vi "Op-Amp Test System.vi"() -> ()   [LabVIEW 2019]
uses:
  <vilib>/Utility/error.llb/DialogType.ctl
  <vilib>/VirtualBench/_DMM Configure Measurement2.vi
  <vilib>/VirtualBench/_PS Configure Voltage Output0.vi
  <vilib>/VirtualBench/_FGEN Configure Standard Waveform14.vi
  <vilib>/VirtualBench/_FGEN Configure Standard Waveform4.vi
  <vilib>/VirtualBench/_MSO Configure Analog Channel28.vi
  <vilib>/VirtualBench/_MSO Configure Timing12.vi
  <vilib>/VirtualBench/_MSO Configure Digital Edge Trigger0.vi
  <vilib>/VirtualBench/_MSO Configure Analog Edge Trigger0.vi
  <vilib>/VirtualBench/_MSO Configure Digital Pattern Trigger0.vi
  <vilib>/VirtualBench/_MSO Configure Analog Channel29.vi
  <vilib>/VirtualBench/VirtualBench.lvlib
  <vilib>/DigilentWF/DigilentWF.lvlib
panel:
  out "测试进度":u8(slide)=100 caption="Testing..." scale=0.0..100.0
  in  "开始测试":bool caption="Start"
  out "Slew Rate(V/us)":dbl=0.5925925925925918 format="%#.2f"
  out "Iin+(mA)":dbl=0.032890531941645075 format="%#.2g"
  out "Voffset(mV)":dbl=0.00017364742031570723 format="%#.2f"
  out "Iin-(mA)":dbl=0.032890531941645075 format="%#.2g"
  in  "图表选项卡":enum32{"Time Domain", "Frequency Domain"}(tab)
  out "Time Domain":waveform(dbl)(graph)={"t0"=timestamp(3648703829.272387 s since 1904-01-01), "dt"=5e-06, "Y"=[1.4814814814814814, 1.522633744855967, 1.522633744855967, 1.522633744855967, 1.522633744855967, -1.4814814814814814, -1.4814814814814814, -1.4814814814814814, -1.4814814814814814, -1.4814814814814814, 1.4814814814814814, 1.4814814814814814, 1.522633744855967, 1.522633744855967, 1.522633744855967, -1.4814814814814814, -1.4814814814814814, -1.4814814814814814, -1.522633744855967, -1.4814814814814814, 1.4814814814814814, 1.4814814814814814, 1.522633744855967, 1.522633744855967, 1.4814814814814814, -1.4814814814814814, -1.4814814814814814, -1.4814814814814814, -1.4814814814814814, -1.4814814814814814, 1.522633744855967, 1.4814814814814814, 1.522633744855967, 1.4814814814814814, 1.522633744855967, -1.4814814814814814, -1.4814814814814814, -1.4814814814814814, -1.4814814814814814, -1.4814814814814814, 1.4814814814814814, 1.522633744855967, 1.522633744855967, 1.522633744855967, 1.4814814814814814, -1.4814814814814814, -1.4814814814814814, -1.4814814814814814, -1.4814814814814814, -1.4814814814814814, 1.522633744855967], "attributes"=variant("NI_ChannelName"=variant(string "mso/1"), "NI_UnitDescription"=variant(string "Volts"))}
  out "Amplitude-frequency":cluster{dbl[], dbl[]}(graph)={[1000.0, 50000.0, 100000.0, 150000.0, 200000.0, 250000.0, 300000.0, 350000.0, 400000.0, 450000.0, 500000.0, 550000.0, 600000.0, 650000.0, 700000.0, 750000.0, 800000.0, 850000.0, 900000.0, 950000.0, 1000000.0], [-0.043499224382493214, -0.07910564758937852, -0.05855677171822875, -0.12520052009093197, -0.0701265456021912, -0.03557595242825849, -0.039394402754777826, 0.019459305615298683, -0.20860878085057782, -0.6531346266811084, -1.6767532340802709, -2.545389095285617, -3.45499166219188, -4.165947530618234, -5.023851452790434, -5.691370407236383, -6.452267174495198, -6.919081220388349, -7.501631061654676, -8.082809544588587, -8.419860804310309]} caption="Amplitude-frequency characteristic"
  out "PSRR(dB)":dbl=139.0596904318624 format="%#.1f"
  out "KCMRR(dB)":dbl=128.17369955860022 format="%#.1f"
  out "Iin_mean(mA)":dbl=0.032890531941645075 format="%#.2g"
  out "Iin_bias(mA)":dbl format="%#.5g"
  out "K0(dB)":dbl=131.53455047796112 format="%#.1f"
  in  "测试参数选项卡":T1(tab)=enum."Slew Rate"
  in  "Current PWS":T2={"PWS Channel"="VB8012-3126A15/ps/+25V", "Voltage Level (V)"=10.0, "Current Limit (A)"=0.05} {"Voltage Level (V)" min=0.0 max=12.0}
  in  "DC Offset(V)":dbl=1.0 caption="DC Offset" format="%#_13g"
  in  "Waveform Function":enum16{"Sine", "Square", "Triangle/Ramp", "DC"}(ring)=enum."DC"
  in  "CMRR PWS 2":T3={"PWS Channel 2"="VB8012-3126A15/ps/-25V", "Voltage Level (V)"=[-9.5, -8.5], "Current Limit (A)"=0.05} {"Voltage Level (V)" min=-12.0 max=0.0}
  in  "CMRR PWS1":T4={"PWS Channel 1"="VB8012-3126A15/ps/+25V", "Voltage Level (V)"=[9.5, 10.5], "Current Limit (A)"=0.05} {"Voltage Level (V)" min=0.0 max=12.0}
  in  "PSRR PWS":T5={"PWS Channel"="VB8012-3126A15/ps/+25V", "Voltage Level (V)"=[9.5, 10.0], "Current Limit (A)"=0.05} {"Voltage Level (V)" min=0.0 max=12.0}
  in  "Slew Rate PWS":T2={"PWS Channel"="VB8012-3126A15/ps/+25V", "Voltage Level (V)"=10.0, "Current Limit (A)"=0.05} {"Voltage Level (V)" min=0.0 max=12.0}
  in  "Frequency":dbl=20000.0 format="%#_13g"
  in  "Slewrate Waveform":enum16{"Sine", "Square", "Triangle/Ramp", "DC"}(ring)=enum."Square" caption="Waveform Function"
  in  "Amplitude":dbl=3.0 format="%#_13g"
  in  "DC Offset":dbl format="%#_13g"
  in  "Channel":tag="VB8012-3126A15/mso/1"
  in  "Vertical Range":dbl=3.0 format="%#_13g"
  in  "Trigger Type":T6(tab)
  in  "Digital Trigger Source":tag="mso/d0" caption="Trigger Source (no change)"
  in  "Edge":i32(ring) caption="Trigger Slope (no change)" items=["Rising", "Falling", "Either"]
  in  "Level (V)":dbl=0.4 format="%0.2f"
  in  "Hysteresis (V)":dbl=0.17
  in  "Analog Trigger Source":tag="VB8012-3126A15/mso/1" caption="Trigger Source (no change)"
  in  "Slope":i32(ring) caption="Trigger Slope (no change)" items=["Rising", "Falling", "Either"]
  in  "Pattern Trigger Source":tag="mso/d0:7" caption="Trigger Source (no change)"
  in  "Trigger Pattern":string="1R0XX1X0" caption="Trigger Pattern (no change)"
  in  "BW PWS":T2={"PWS Channel"="VB8012-3126A15/ps/+25V", "Voltage Level (V)"=10.0, "Current Limit (A)"=0.05} {"Voltage Level (V)" min=0.0 max=12.0}
  in  "Slewrate Waveform":enum16{"Sine", "Square", "Triangle/Ramp", "DC"}(ring) caption="Waveform Function"
  in  "Amplitude":dbl=2.0 format="%#_13g"
  in  "DC Offset":dbl format="%#_13g"
  in  "Vertical Range":dbl=3.0 format="%#_13g"
  in  "Channel":tag="VB8012-3126A15/mso/1"
  in  "Trigger Type":T6(tab)
  in  "Digital Trigger Source":tag="mso/d0" caption="Trigger Source (no change)"
  in  "Edge":i32(ring) caption="Trigger Slope (no change)" items=["Rising", "Falling", "Either"]
  in  "Analog Trigger Source":tag="mso/1" caption="Trigger Source (no change)"
  in  "Slope":i32(ring) caption="Trigger Slope (no change)" items=["Rising", "Falling", "Either"]
  in  "Level (V)":dbl format="%0.2f"
  in  "Hysteresis (V)":dbl=0.17
  in  "Pattern Trigger Source":tag="mso/d0:7" caption="Trigger Source (no change)"
  in  "Trigger Pattern":string="1R0XX1X0" caption="Trigger Pattern (no change)"
  in  "测试机台选择":tag="VB8012-3126A15"
  # "基于IECUBE-3839的运放自动化测试程序"
  # "硬件配置"
  # "DUT测试参数"
  # "设备选择"
  # "DUT测试结果"
  # "电源配置"
  # "函数发生器配置"
  # "电源配置"
  # "电源配置"
  # "电源配置"
  # "函数发生器配置"
  # "逻辑分析仪配置"
  # "Triggers immediately after MSO Run VI executes."
  # "电源配置"
  # "函数发生器配置"
  # "逻辑分析仪配置"
  # "Triggers immediately after MSO Run VI executes."
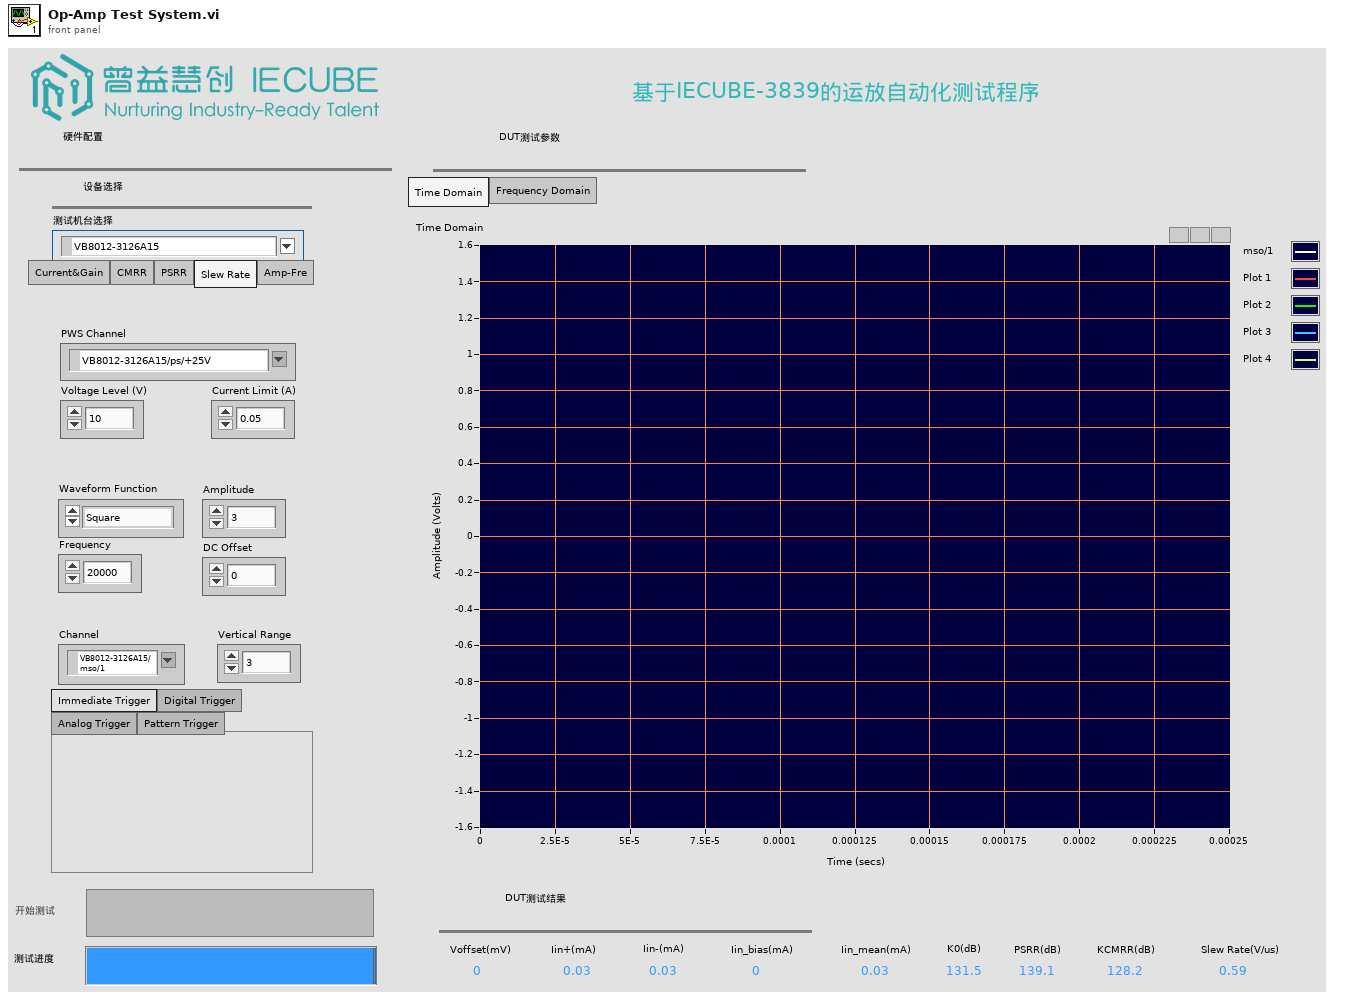
[diagram p1: front panel]
types:
  T1 = enum32{"Current&Gain", "CMRR", "PSRR", "Slew Rate", "Amp-Fre"}
  T2 = cluster{"PWS Channel":tag, "Voltage Level (V)":dbl, "Current Limit (A)":dbl}
  T3 = cluster{"PWS Channel 2":tag, "Voltage Level (V)":dbl[], "Current Limit (A)":dbl}
  T4 = cluster{"PWS Channel 1":tag, "Voltage Level (V)":dbl[], "Current Limit (A)":dbl}
  T5 = cluster{"PWS Channel":tag, "Voltage Level (V)":dbl[], "Current Limit (A)":dbl}
  T6 = enum32{"Immediate Trigger", "Digital Trigger", "Analog Trigger", "Pattern Trigger"}
  T7 = typedef "测试参数.ctl" = enum16{"Leakage Current", "Gain", "CMRR", "PSRR", "Slew Rate", "Amplitude-Frequency"}
  T8 = typedef "DialogType.ctl" = u16
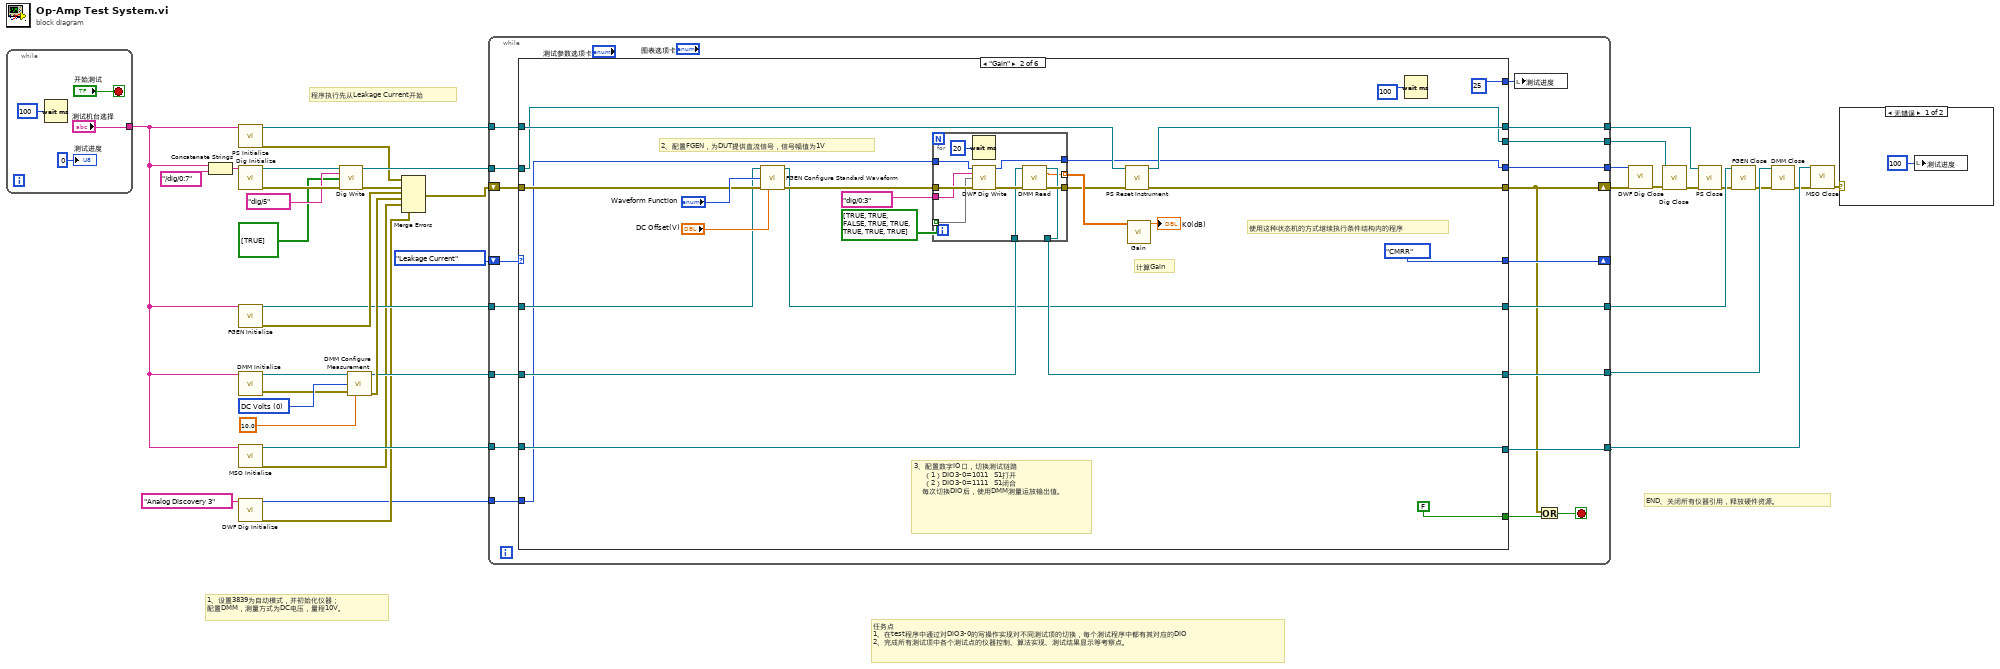
[diagram p0: block diagram]
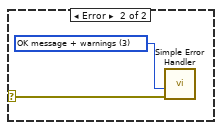
[diagram p2: hidden frame]
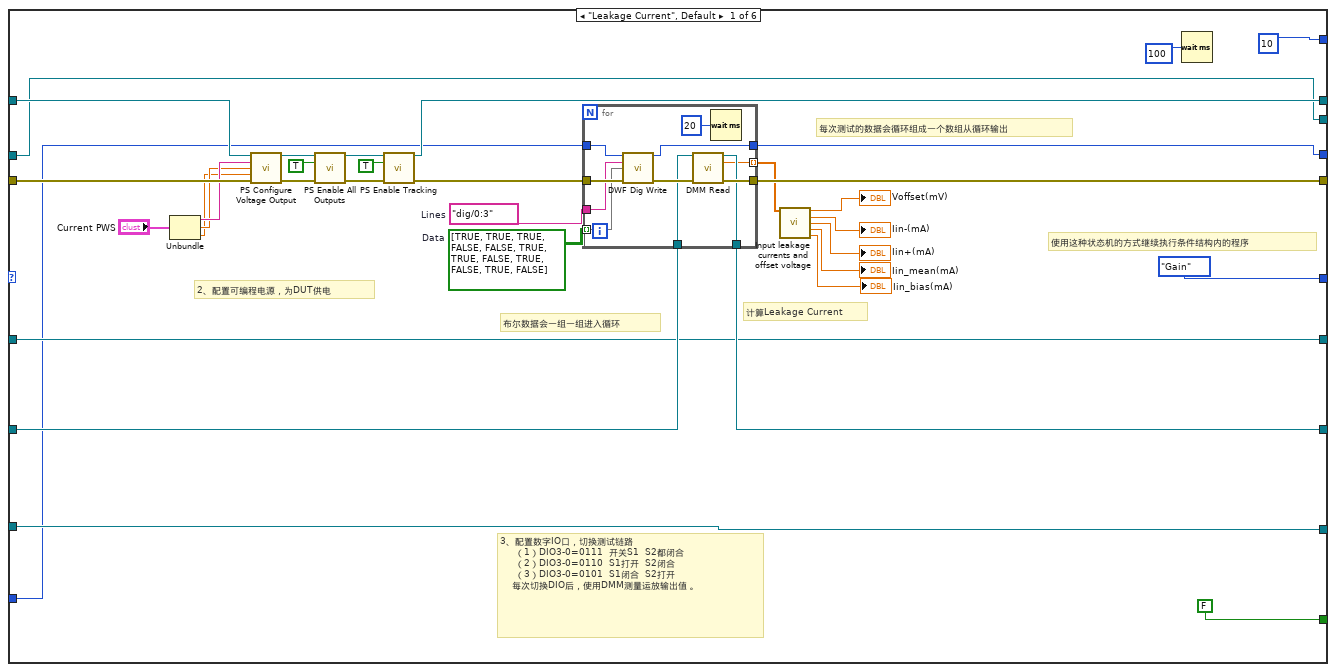
[diagram p3: hidden frame]
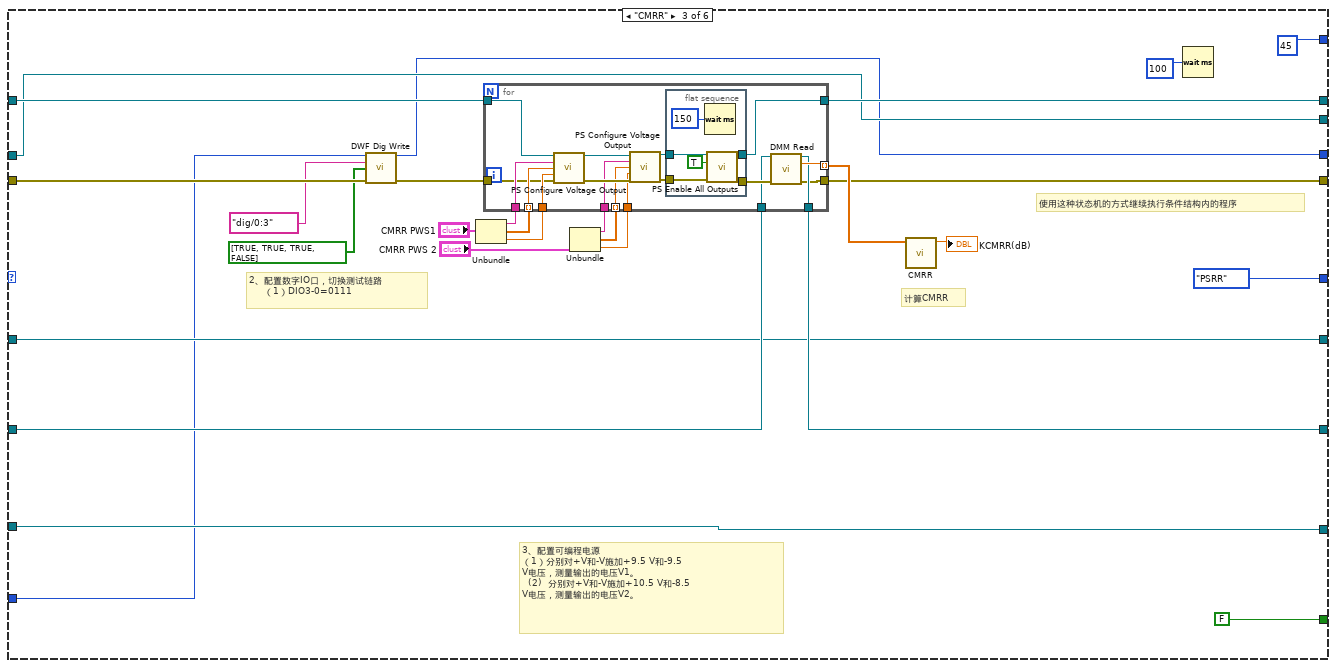
[diagram p4: hidden frame]
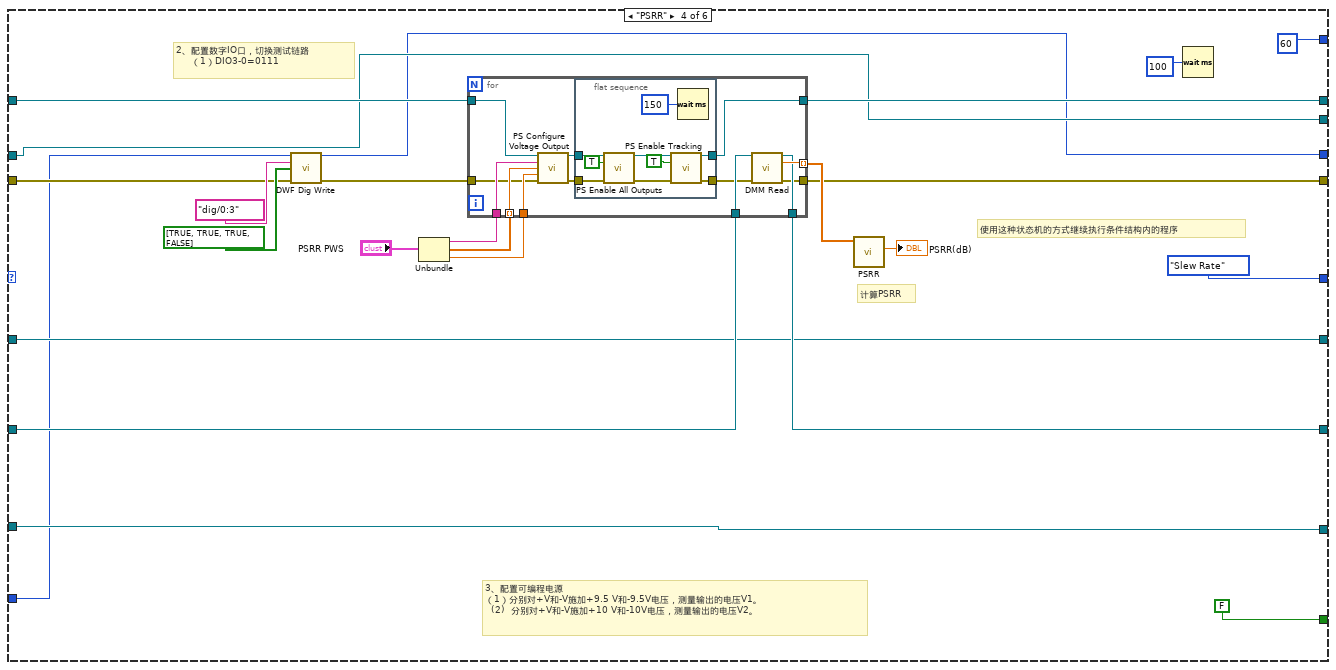
[diagram p5: hidden frame]
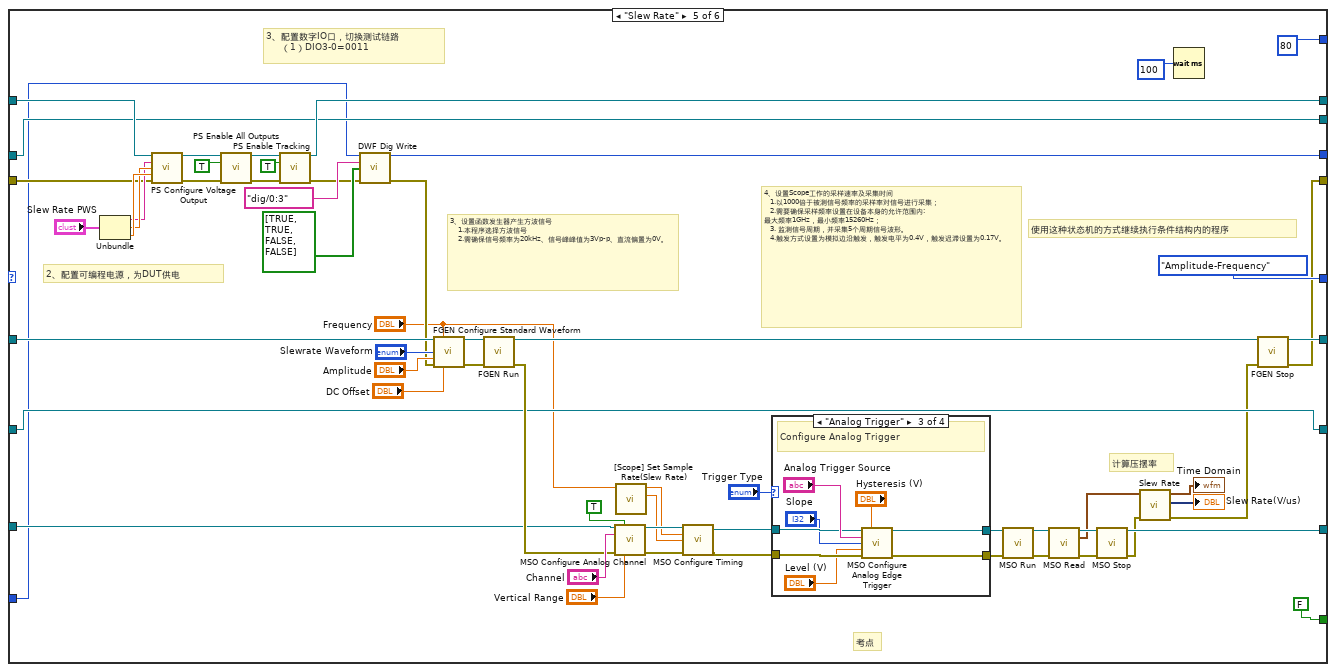
[diagram p6: hidden frame]
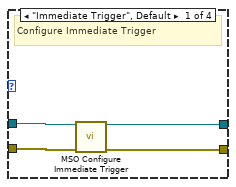
[diagram p7: hidden frame]
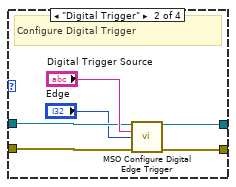
[diagram p8: hidden frame]
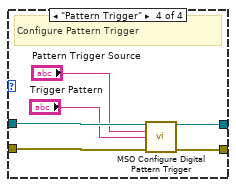
[diagram p9: hidden frame]
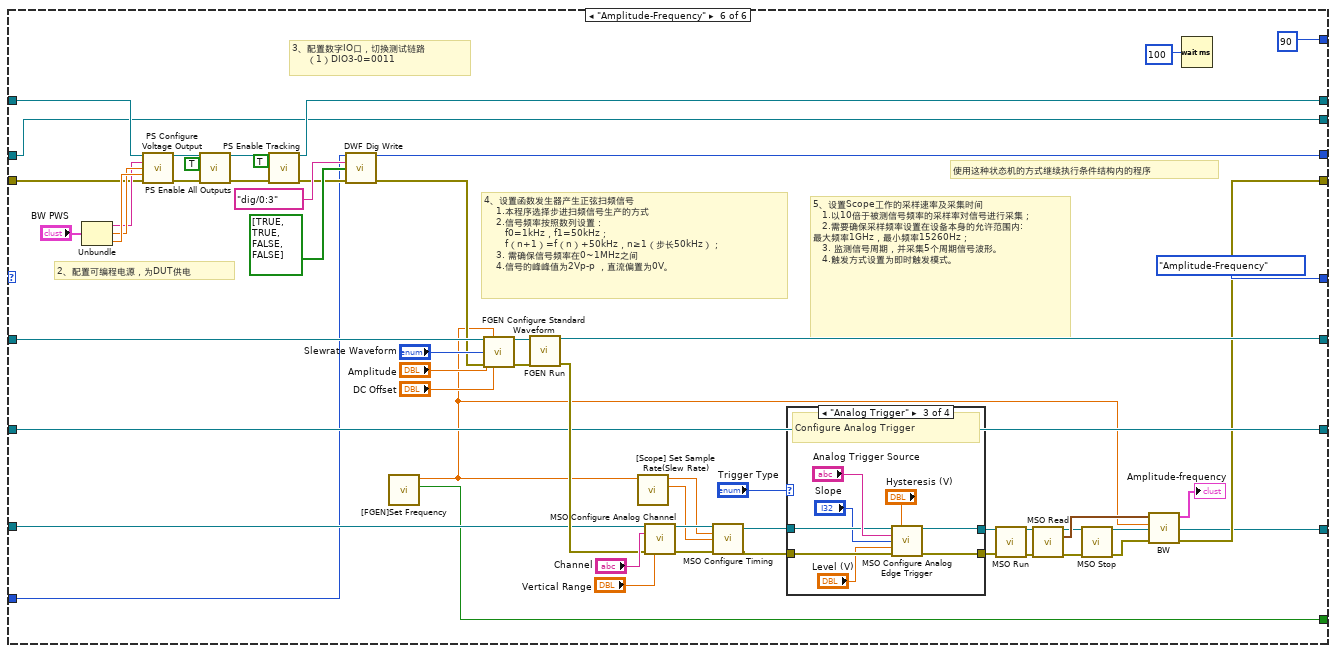
[diagram p10: hidden frame]
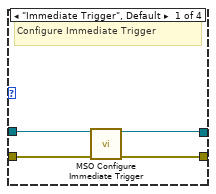
[diagram p11: hidden frame]
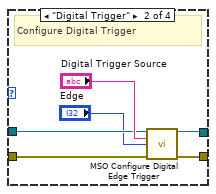
[diagram p12: hidden frame]
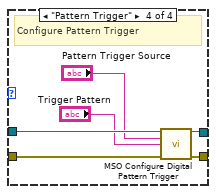
[diagram p13: hidden frame]
diagram:
  w29 = 0 items=["DC Volts", "AC Volts", "DC Current", "AC Current", "Resistance", "Diode"] ("Function")
  # "程序执行先从Leakage Current开始"
  # "任务点\n1、在test程序中通过对DIO3-0的写操作实现对不同测试项的切换，每个测试程序中都有其对应的DIO\n2、完成所有测试项中各个测试点的仪器控制、算法实现、测试结果显示等考察点。"
  # "END、关闭所有仪器引用，释放硬件资源。"
  # "1、设置3839为自动模式，并初始化仪器；\n配置DMM，测量方式为DC电压，量程10V。"
  n1 = while {
    tunnel: ["测试机台选择"] -> w16
    stop <- "开始测试" stop-if-true
    n2 = Wait (ms)(milliseconds to wait=u32 100 ("等待时间（毫秒）")) -> ()  [unwired: 1 out]
    "测试进度" <- u8 0 ("测试进度")
  }
  n3 = Concatenate Strings(w16, "/dig/0:7" ("字符串")) -> (w34:string)
  n4 = call <vilib>:"PS Initialize.vi"("Device Name"=w16) -> ("Instrument Handle Out"=w33:refnum<k21>, "Error Out"=w13:errorcluster)  [unwired: 13 in]
  n5 = call <vilib>:"Dig Initialize.vi"("Lines"=w34) -> ("Instrument Handle Out"=w39:refnum<k21>, "Error Out"=w38:errorcluster)  [unwired: 13 in]
  n6 = call <vilib>:"FGEN Initialize.vi"("Device Name"=w16) -> ("Instrument Handle Out"=w22:refnum<k21>, "Error Out"=w23:errorcluster)  [unwired: 13 in]
  n7 = call <vilib>:"DMM Initialize.vi"("Device Name"=w16) -> ("Instrument Handle Out"=w27:refnum<k21>, "Error Out"=w28:errorcluster)  [unwired: 13 in]
  n8 = call <vilib>:"MSO Initialize.vi"("Device Name"=w16) -> ("Instrument Handle Out"=w15:refnum<k21>, "Error Out"=w14:errorcluster)  [unwired: 13 in]
  n9 = call <vilib>:"DWF Dig Initialize.vi"("Device Name/Lines"="Analog Discovery 3") -> ("Instrument Handle Out"=w4:u32, "Error Out"=w5:errorcluster)  [unwired: 13 in]
  n10 = call <vilib>:"Dig Write.vi"("Instrument Handle In"=w39, "Lines"=tag "dig/5", "Data"=bool[] [TRUE], "Error In"=w38) -> ("Instrument Handle Out"=w32:refnum<k21>, "Error Out"=w12:errorcluster)  [unwired: 10 in]
  n11 = call-poly <vilib>:"DMM Configure Measurement.vi"("Instrument Handle In"=w27, "Function"=w29, "Error In"=w28, "Manual Range"=10.0) -> ("Instrument Handle Out"=w25:refnum<k21>, "Error Out"=w26:errorcluster)  [unwired: 10 in]
  n12 = Merge Errors(w13, w12, w23, w26, w14, w5) -> (w30:errorcluster)
  n13 = while {
    tunnel: w32 -> [w60]
    tunnel: w33 -> [w58]
    shift-right: [w59] -> _
    shift-left: 测试参数."Leakage Current" -> [w62]
    tunnel: w25 -> [w57]
    tunnel: [w56] -> w19
    shift-right: [w48] -> w2
    shift-left: w30 -> [w61]
    tunnel: [w55] -> w21
    tunnel: [w54] -> w20
    tunnel: w22 -> [w53]
    tunnel: [w52] -> w18
    tunnel: [w51] -> w17
    tunnel: w15 -> [w50]
    tunnel: w4 -> [w45]
    tunnel: [w44] -> w1
    stop <- w46 stop-if-true
    n14 = case shown="\"Gain\"" w62 {
      tunnel: w61 -> [w82 w122 w149 w198 w263 w344]
      tunnel: w60 -> [w65 w110 w145 w197 w243 w326]
      tunnel: [测试参数."Gain" 测试参数."CMRR" 测试参数."PSRR" 测试参数."Slew Rate" 测试参数."Amplitude-Frequency" 测试参数."Amplitude-Frequency"] -> w59
      tunnel: w58 -> [w80 w113 w167 w215 w262 w343]
      tunnel: w57 -> [w92 w124 w164 w212 w249 w362]
      tunnel: [w65 w110 w145 w197 w243 w326] -> w56
      tunnel: [w90 w114 w153 w204 w258 w340] -> w48
      tunnel: [w89 w123 w163 w211 w249 w362] -> w55
      tunnel: [w76 w112 w150 w203 w254 w341] -> w54
      tunnel: w53 -> [w75 w121 w162 w210 w281 w361]
      tunnel: [w75 w119 w162 w210 w259 w360] -> w52
      tunnel: [w74 w118 w161 w209 w278 w331] -> w51
      tunnel: w50 -> [w74 w118 w161 w209 w280 w359]
      tunnel: [FALSE FALSE FALSE FALSE FALSE w328] -> w47
      tunnel: [10 25 45 60 80 90] -> w49
      tunnel: w45 -> [w63 w108 w144 w195 w242 w325]
      tunnel: [w64 w109 w143 w196 w241 w324] -> w44
      frame "Leakage Current", Default {
        w91 = tag "dig/0:3"  # Lines
        w96 = bool[][] [[TRUE, TRUE, TRUE, FALSE], [FALSE, TRUE, TRUE, FALSE], [TRUE, FALSE, TRUE, FALSE]]  # Data
        # "计算Leakage Current"
        # "使用这种状态机的方式继续执行条件结构内的程序"
        # "每次测试的数据会循环组成一个数组从循环输出"
        # "布尔数据会一组一组进入循环"
        # "3、配置数字IO口，切换测试链路\n     （1）DIO3-0=0111  开关S1  S2都闭合\n     （2）DIO3-0=0110  S1打开  S2闭合 \n     （3）DIO3-0=0101  S1闭合  S2打开\n    每次切换DIO后，使用DMM测量运放输出值 。"
        # "2、配置可编程电源，为DUT供电"
        n15 = Unbundle("Current PWS") -> ("PWS Channel"=w79:tag, "Voltage Level (V)"=w78:dbl, "Current Limit (A)"=w77:dbl)
        n16 = call-poly <vilib>:"PS Configure Voltage Output.vi"("Instrument Handle In"=w80, "Channel"=w79, "Voltage Level"=w78, "Current Limit"=w77, "Error In"=w82) -> ("Instrument Handle Out"=w88:refnum<k21>, "Error Out"=w87:errorcluster)  [unwired: 9 in]
        n17 = call <vilib>:"PS Enable All Outputs.vi"("Instrument Handle In"=w88, "Enable Outputs"=TRUE, "Error In"=w87) -> ("Instrument Handle Out"=w85:refnum<k21>, "Error Out"=w84:errorcluster)  [unwired: 11 in]
        n18 = call <vilib>:"PS Enable Tracking.vi"("Instrument Handle In"=w85, "Enable Tracking"=TRUE, "Error In"=w84) -> ("Instrument Handle Out"=w76:refnum<k21>, "Error Out"=w81:errorcluster)  [unwired: 11 in]
        n19 = for {
          tunnel: w81 -> [w107]
          tunnel: [w106] -> w90
          tunnel: [w105] -> w89
          tunnel: w96 -> [w104] mode=indexing
          tunnel: [w103] -> w71 mode=indexing
          tunnel: w92 -> [w101]
          tunnel: w63 -> [w100]
          tunnel: [w99] -> w64
          tunnel: w91 -> [w98]
          n20 = call <vilib>:"DWF Dig Write.vi"("Instrument Handle In"=w100, "Lines"=w98, "Data"=w104, "Error In"=w107) -> ("Instrument Handle Out"=w99:u32, "Error Out"=w102:errorcluster)  [unwired: 10 in]
          n21 = call <vilib>:"DMM Read.vi"("Instrument Handle In"=w101, "Error In"=w102) -> ("Instrument Handle Out"=w105:refnum<k21>, "Measurement"=w103:dbl, "Error Out"=w106:errorcluster)  [unwired: 11 in]
          n22 = Wait (ms)(milliseconds to wait=u32 20 ("等待时间（毫秒）")) -> ()  [unwired: 1 out]
        }
        n23 = call "Input leakage currents and offset voltage.vi"("数组输入"=w71) -> ("Voffset"=→"Voffset(mV)":dbl, "Iin-"=→"Iin-(mA)":dbl, "Iin+"=→"Iin+(mA)":dbl, "Iin_mean"=→"Iin_mean(mA)":dbl, "Iin_bias"=→"Iin_bias(mA)":dbl)  [unwired: 10 in]
        n24 = Wait (ms)(milliseconds to wait=u32 100 ("等待时间（毫秒）")) -> ()  [unwired: 1 out]
      }
      frame "Gain" {
        # "计算Gain"
        # "使用这种状态机的方式继续执行条件结构内的程序"
        # "2、配置FGEN，为DUT提供直流信号，信号幅值为1V"
        # "3、配置数字IO口，切换测试链路\n     （1）DIO3-0=1011   S1打开\n     （2）DIO3-0=1111   S1闭合\n    每次切换DIO后，使用DMM测量运放输出值。"
        n25 = call-poly <vilib>:"FGEN Configure Standard Waveform.vi"("Instrument Handle In"=w121, "Waveform Function"="Waveform Function", "Error In"=w122, "DC Offset"="DC Offset(V)") -> ("Instrument Handle Out"=w119:refnum<k21>, "Error Out"=w127:errorcluster)  [unwired: 10 in]
        n26 = for {
          tunnel: w127 -> [w142]
          tunnel: [w141] -> w115
          tunnel: [w140] -> w123
          tunnel: bool[][] [[TRUE, TRUE, FALSE, TRUE], [TRUE, TRUE, TRUE, TRUE]] ("Data") -> [w139] mode=indexing
          tunnel: [w138] -> w130 mode=indexing
          tunnel: w124 -> [w136]
          tunnel: tag "dig/0:3" ("Lines") -> [w134]
          tunnel: [w133] -> w109
          tunnel: w108 -> [w132]
          n27 = Wait (ms)(milliseconds to wait=u32 20 ("等待时间（毫秒）")) -> ()  [unwired: 1 out]
          n28 = call <vilib>:"DWF Dig Write.vi"("Instrument Handle In"=w132, "Lines"=w134, "Data"=w139, "Error In"=w142) -> ("Instrument Handle Out"=w133:u32, "Error Out"=w137:errorcluster)  [unwired: 10 in]
          n29 = call <vilib>:"DMM Read.vi"("Instrument Handle In"=w136, "Error In"=w137) -> ("Instrument Handle Out"=w140:refnum<k21>, "Measurement"=w138:dbl, "Error Out"=w141:errorcluster)  [unwired: 11 in]
        }
        n30 = call <vilib>:"PS Reset Instrument.vi"("Instrument Handle In"=w113, "Error In"=w115) -> ("Instrument Handle Out"=w112:refnum<k21>, "Error Out"=w114:errorcluster)  [unwired: 12 in]
        n31 = call "Gain.vi"("数组"=w130) -> ("K0"=→"K0(dB)":dbl)  [unwired: 10 in]
        n32 = Wait (ms)(milliseconds to wait=u32 100 ("等待时间（毫秒）")) -> ()  [unwired: 1 out]
      }
      frame "CMRR" {
        # "计算CMRR"
        # "使用这种状态机的方式继续执行条件结构内的程序"
        # "3、配置可编程电源\n（1）分别对+V和-V施加+9.5 V和-9.5 V电压，测量输出的电压V1。\n  (2)  分别对+V和-V施加+10.5 V和-8.5 V电压，测量输出的电压V2。"
        # "2、配置数字IO口，切换测试链路\n     （1）DIO3-0=0111"
        n33 = call <vilib>:"DWF Dig Write.vi"("Instrument Handle In"=w144, "Lines"=tag "dig/0:3", "Data"=bool[] [TRUE, TRUE, TRUE, FALSE], "Error In"=w149) -> ("Instrument Handle Out"=w143:u32, "Error Out"=w148:errorcluster)  [unwired: 10 in]
        n34 = Unbundle("CMRR PWS1") -> ("PWS Channel 1"=w168:tag, "Voltage Level (V)"=w169:dbl[], "Current Limit (A)"=w170:dbl)
        n35 = Unbundle("CMRR PWS 2") -> ("PWS Channel 2"=w156:tag, "Voltage Level (V)"=w155:dbl[], "Current Limit (A)"=w154:dbl)
        n36 = for {
          tunnel: w170 -> [w188]
          tunnel: w169 -> [w187] mode=indexing
          tunnel: w167 -> [w186]
          tunnel: w168 -> [w185]
          tunnel: w148 -> [w184]
          tunnel: w164 -> [w182]
          tunnel: [w181] -> w166 mode=indexing
          tunnel: [w180] -> w163
          tunnel: [w179] -> w153
          tunnel: w156 -> [w174]
          tunnel: w155 -> [w173] mode=indexing
          tunnel: w154 -> [w172]
          tunnel: [w171] -> w150
          n37 = call-poly <vilib>:"PS Configure Voltage Output.vi"("Instrument Handle In"=w186, "Channel"=w185, "Voltage Level"=w187, "Current Limit"=w188, "Error In"=w184) -> ("Instrument Handle Out"=w178:refnum<k21>, "Error Out"=w177:errorcluster)  [unwired: 9 in]
          n38 = call-poly <vilib>:"PS Configure Voltage Output.vi"("Instrument Handle In"=w178, "Channel"=w174, "Voltage Level"=w173, "Current Limit"=w172, "Error In"=w177) -> ("Instrument Handle Out"=w175:refnum<k21>, "Error Out"=w176:errorcluster)  [unwired: 9 in]
          n39 = flat-sequence {
            tunnel: [w193] -> w183
            tunnel: w176 -> [w192]
            tunnel: w175 -> [w191]
            tunnel: [w190] -> w171
            frame #0 {
              n40 = Wait (ms)(milliseconds to wait=u32 150 ("等待时间（毫秒）")) -> ()  [unwired: 1 out]
              n41 = call <vilib>:"PS Enable All Outputs.vi"("Instrument Handle In"=w191, "Enable Outputs"=TRUE ("Enable Output"), "Error In"=w192) -> ("Instrument Handle Out"=w190:refnum<k21>, "Error Out"=w193:errorcluster)  [unwired: 11 in]
            }
          }
          n42 = call <vilib>:"DMM Read.vi"("Instrument Handle In"=w182, "Error In"=w183) -> ("Instrument Handle Out"=w180:refnum<k21>, "Measurement"=w181:dbl, "Error Out"=w179:errorcluster)  [unwired: 11 in]
        }
        n43 = call "CMRR.vi"("数组"=w166) -> ("KCMRR"=→"KCMRR(dB)":dbl)  [unwired: 10 in]
        n44 = Wait (ms)(milliseconds to wait=u32 100 ("等待时间（毫秒）")) -> ()  [unwired: 1 out]
      }
      frame "PSRR" {
        # "计算PSRR"
        # "使用这种状态机的方式继续执行条件结构内的程序"
        # "3、配置可编程电源\n（1）分别对+V和-V施加+9.5 V和-9.5V电压，测量输出的电压V1。\n  (2)  分别对+V和-V施加+10 V和-10V电压，测量输出的电压V2。"
        # "2、配置数字IO口，切换测试链路\n     （1）DIO3-0=0111"
        n45 = call <vilib>:"DWF Dig Write.vi"("Instrument Handle In"=w195, "Lines"=tag "dig/0:3", "Data"=bool[] [TRUE, TRUE, TRUE, FALSE], "Error In"=w198) -> ("Instrument Handle Out"=w196:u32, "Error Out"=w199:errorcluster)  [unwired: 10 in]
        n46 = Unbundle("PSRR PWS") -> ("PWS Channel"=w216:tag, "Voltage Level (V)"=w217:dbl[], "Current Limit (A)"=w218:dbl)
        n47 = for {
          tunnel: w218 -> [w231]
          tunnel: w217 -> [w230] mode=indexing
          tunnel: w215 -> [w229]
          tunnel: w216 -> [w228]
          tunnel: w199 -> [w227]
          tunnel: w212 -> [w226]
          tunnel: [w225] -> w214 mode=indexing
          tunnel: [w224] -> w211
          tunnel: [w223] -> w204
          tunnel: [w220] -> w203
          n48 = call-poly <vilib>:"PS Configure Voltage Output.vi"("Instrument Handle In"=w229, "Channel"=w228, "Voltage Level"=w230, "Current Limit"=w231, "Error In"=w227) -> ("Instrument Handle Out"=w222:refnum<k21>, "Error Out"=w221:errorcluster)  [unwired: 9 in]
          n49 = flat-sequence {
            tunnel: w222 -> [w239]
            tunnel: w221 -> [w238]
            tunnel: [w235] -> w220
            tunnel: [w234] -> w219
            frame #0 {
              n50 = call <vilib>:"PS Enable All Outputs.vi"("Instrument Handle In"=w239, "Enable Outputs"=TRUE ("Enable Output"), "Error In"=w238) -> ("Instrument Handle Out"=w236:refnum<k21>, "Error Out"=w237:errorcluster)  [unwired: 11 in]
              n51 = call <vilib>:"PS Enable Tracking.vi"("Instrument Handle In"=w236, "Enable Tracking"=TRUE, "Error In"=w237) -> ("Instrument Handle Out"=w235:refnum<k21>, "Error Out"=w234:errorcluster)  [unwired: 11 in]
              n52 = Wait (ms)(milliseconds to wait=u32 150 ("等待时间（毫秒）")) -> ()  [unwired: 1 out]
            }
          }
          n53 = call <vilib>:"DMM Read.vi"("Instrument Handle In"=w226, "Error In"=w219) -> ("Instrument Handle Out"=w224:refnum<k21>, "Measurement"=w225:dbl, "Error Out"=w223:errorcluster)  [unwired: 11 in]
        }
        n54 = call "PSRR.vi"("数组"=w214) -> ("PSRR"=→"PSRR(dB)":dbl)  [unwired: 10 in]
        n55 = Wait (ms)(milliseconds to wait=u32 100 ("等待时间（毫秒）")) -> ()  [unwired: 1 out]
      }
      frame "Slew Rate" {
        # "计算压摆率"
        # "使用这种状态机的方式继续执行条件结构内的程序"
        # "考点"
        # "3、配置数字IO口，切换测试链路\n     （1）DIO3-0=0011"
        # "4、设置Scope工作的采样速率及采集时间\n   1.以1000倍于被测信号频率的采样率对信号进行采集；\n   2.需要确保采样频率设置在设备本身的允许范围内: 最大频率1GHz，最小频率15260Hz；\n   3. 监测信号周期，并采集5个周期信号波形。\n   4.触发方式设置为模拟边沿触发，触发电平为0.4V，触发迟滞设置为0.17V。"
        # "3、设置函数发生器产生方波信号\n    1.本程序选择方波信号\n    2.需确保信号频率为20kHz、信号峰峰值为3Vp-p、直流偏置为0V。"
        # "2、配置可编程电源，为DUT供电"
        n56 = Unbundle("Slew Rate PWS") -> ("PWS Channel"=w268:tag, "Voltage Level (V)"=w269:dbl, "Current Limit (A)"=w270:dbl)
        n57 = call-poly <vilib>:"PS Configure Voltage Output.vi"("Instrument Handle In"=w262, "Channel"=w268, "Voltage Level"=w269, "Current Limit"=w270, "Error In"=w263) -> ("Instrument Handle Out"=w265:refnum<k21>, "Error Out"=w266:errorcluster)  [unwired: 9 in]
        n58 = call <vilib>:"PS Enable All Outputs.vi"("Instrument Handle In"=w265, "Enable Outputs"=TRUE, "Error In"=w266) -> ("Instrument Handle Out"=w255:refnum<k21>, "Error Out"=w267:errorcluster)  [unwired: 11 in]
        n59 = call <vilib>:"PS Enable Tracking.vi"("Instrument Handle In"=w255, "Enable Tracking"=TRUE, "Error In"=w267) -> ("Instrument Handle Out"=w254:refnum<k21>, "Error Out"=w256:errorcluster)  [unwired: 11 in]
        n60 = call <vilib>:"DWF Dig Write.vi"("Instrument Handle In"=w242, "Lines"=tag "dig/0:3", "Data"=bool[] [TRUE, TRUE, FALSE, FALSE], "Error In"=w256) -> ("Instrument Handle Out"=w241:u32, "Error Out"=w271:errorcluster)  [unwired: 10 in]
        n61 = call-poly <vilib>:"FGEN Configure Standard Waveform.vi"("Instrument Handle In"=w281, "Frequency"="Frequency", "Waveform Function"="Slewrate Waveform", "Amplitude"="Amplitude", "Error In"=w271, "DC Offset"="DC Offset") -> ("Instrument Handle Out"=w295:refnum<k21>, "Error Out"=w296:errorcluster)  [unwired: 8 in]
        n62 = call <vilib>:"FGEN Run.vi"("Instrument Handle In"=w295, "Error In"=w296) -> ("Instrument Handle Out"=w260:refnum<k21>, "Error Out"=w291:errorcluster)  [unwired: 12 in]
        n63 = call-poly <vilib>:"MSO Configure Analog Channel.vi"("Instrument Handle In"=w280, "Enable Channel"=TRUE, "Channel"="Channel", "Error In"=w291, "Vertical Range"="Vertical Range") -> ("Instrument Handle Out"=w288:refnum<k21>, "Error Out"=w289:errorcluster)  [unwired: 9 in]
        n64 = call "[Scope] Set Sample Rate(Slew Rate).vi"("Frequency"="Frequency") -> ("Acquistion Time"=w244:dbl, "Sample Rate"=w245:dbl)  [unwired: 9 in]
        n65 = call-poly <vilib>:"MSO Configure Timing.vi"("Instrument Handle In"=w288, "Sample Rate"=w245, "Acquisition Time (s)"=w244, "Error In"=w289) -> ("Instrument Handle Out"=w287:refnum<k21>, "Error Out"=w286:errorcluster)  [unwired: 10 in]
        n66 = case shown="\"Analog Trigger\"" "Trigger Type" {
          tunnel: w287 -> [w303 w306 w311 w321]
          tunnel: w286 -> [w301 w308 w316 w319]
          tunnel: [w302 w305 w312 w322] -> w284
          tunnel: [w300 w309 w315 w323] -> w285
          frame "Immediate Trigger", Default {
            # "Configure Immediate Trigger"
            n67 = call <vilib>:"MSO Configure Immediate Trigger.vi"("Instrument Handle In"=w303, "Error In"=w301) -> ("Instrument Handle Out"=w302:refnum<k21>, "Error Out"=w300:errorcluster)  [unwired: 12 in]
          }
          frame "Digital Trigger" {
            # "Configure Digital Trigger"
            n68 = call-poly <vilib>:"MSO Configure Digital Edge Trigger.vi"("Instrument Handle In"=w306, "Trigger Source"="Digital Trigger Source", "Trigger Slope"="Edge", "Error In"=w308) -> ("Instrument Handle Out"=w305:refnum<k21>, "Error Out"=w309:errorcluster)  [unwired: 10 in]
          }
          frame "Analog Trigger" {
            # "Configure Analog Trigger"
            n69 = call-poly <vilib>:"MSO Configure Analog Edge Trigger.vi"("Instrument Handle In"=w311, "Trigger Hysteresis"="Hysteresis (V)", "Trigger Source"="Analog Trigger Source", "Trigger Slope"="Slope", "Trigger Level"="Level (V)", "Error In"=w316) -> ("Instrument Handle Out"=w312:refnum<k21>, "Error Out"=w315:errorcluster)  [unwired: 8 in]
          }
          frame "Pattern Trigger" {
            # "Configure Pattern Trigger"
            n70 = call-poly <vilib>:"MSO Configure Digital Pattern Trigger.vi"("Instrument Handle In"=w321, "Trigger Source"="Pattern Trigger Source", "Trigger Pattern"="Trigger Pattern", "Error In"=w319) -> ("Instrument Handle Out"=w322:refnum<k21>, "Error Out"=w323:errorcluster)  [unwired: 10 in]
          }
        }
        n71 = call <vilib>:"MSO Run.vi"("Instrument Handle In"=w284, "Error In"=w285) -> ("Instrument Handle Out"=w276:refnum<k21>, "Error Out"=w275:errorcluster)  [unwired: 12 in]
        n72 = call <vilib>:"MSO Read.vi"("Instrument Handle In"=w276, "Error In"=w275) -> ("Instrument Handle Out"=w282:refnum<k21>, "Analog Waveforms"=w274:waveform(dbl)[], "Error Out"=w277:errorcluster)  [unwired: 8 in, 3 out]
        n73 = call <vilib>:"MSO Stop.vi"("Instrument Handle In"=w282, "Error In"=w277) -> ("Instrument Handle Out"=w278:refnum<k21>, "Error Out"=w248:errorcluster)  [unwired: 12 in]
        n74 = call "Slew Rate.vi"("错误输入（无错误）"=w248, "Analog Waveforms"=w274) -> ("错误输出"=w247:errorcluster, "Dynamic Data"=→"Slew Rate(V/us)":dynamicdata, "waveform"=→"Time Domain":waveform(dbl))  [unwired: 7 in]
        n75 = Wait (ms)(milliseconds to wait=u32 100 ("等待时间（毫秒）")) -> ()  [unwired: 1 out]
        n76 = call <vilib>:"FGEN Stop.vi"("Instrument Handle In"=w260, "Error In"=w247) -> ("Instrument Handle Out"=w259:refnum<k21>, "Error Out"=w258:errorcluster)  [unwired: 12 in]
      }
      frame "Amplitude-Frequency" {
        # "使用这种状态机的方式继续执行条件结构内的程序"
        # "3、配置数字IO口，切换测试链路\n     （1）DIO3-0=0011"
        # "5、设置Scope工作的采样速率及采集时间\n   1.以10倍于被测信号频率的采样率对信号进行采集；\n   2.需要确保采样频率设置在设备本身的允许范围内: 最大频率1GHz，最小频率15260Hz；\n   3. 监测信号周期，并采集5个周期信号波形。\n   4.触发方式设置为即时触发模式。"
        # "4、设置函数发生器产生正弦扫频信号\n    1.本程序选择步进扫频信号生产的方式\n    2.信号频率按照数列设置：\n       f0=1kHz，f1=50kHz；\n       f（n+1）=f（n）+50kHz，n≥1（步长50kHz）；\n    3. 需确保信号频率在0~1MHz之间\n    4.信号的峰峰值为2Vp-p ，直流偏置为0V。"
        # "2、配置可编程电源，为DUT供电"
        n77 = Unbundle("BW PWS") -> ("PWS Channel"=w351:tag, "Voltage Level (V)"=w352:dbl, "Current Limit (A)"=w353:dbl)
        n78 = call-poly <vilib>:"PS Configure Voltage Output.vi"("Instrument Handle In"=w343, "Channel"=w351, "Voltage Level"=w352, "Current Limit"=w353, "Error In"=w344) -> ("Instrument Handle Out"=w347:refnum<k21>, "Error Out"=w348:errorcluster)  [unwired: 9 in]
        n79 = call <vilib>:"PS Enable All Outputs.vi"("Instrument Handle In"=w347, "Enable Outputs"=TRUE, "Error In"=w348) -> ("Instrument Handle Out"=w349:refnum<k21>, "Error Out"=w350:errorcluster)  [unwired: 11 in]
        n80 = call <vilib>:"PS Enable Tracking.vi"("Instrument Handle In"=w349, "Enable Tracking"=TRUE, "Error In"=w350) -> ("Instrument Handle Out"=w341:refnum<k21>, "Error Out"=w342:errorcluster)  [unwired: 11 in]
        n81 = call <vilib>:"DWF Dig Write.vi"("Instrument Handle In"=w325, "Lines"=tag "dig/0:3", "Data"=bool[] [TRUE, TRUE, FALSE, FALSE], "Error In"=w342) -> ("Instrument Handle Out"=w324:u32, "Error Out"=w354:errorcluster)  [unwired: 10 in]
        n82 = call "[FGEN]Set Frequency.vi"() -> ("Freq in range?"=w328:bool, "Frequency"=w327:dbl)  [unwired: 10 in]
        n83 = call-poly <vilib>:"FGEN Configure Standard Waveform.vi"("Instrument Handle In"=w361, "Frequency"=w327, "Waveform Function"="Slewrate Waveform", "Amplitude"="Amplitude", "Error In"=w354, "DC Offset"="DC Offset") -> ("Instrument Handle Out"=w374:refnum<k21>, "Error Out"=w375:errorcluster)  [unwired: 8 in]
        n84 = call <vilib>:"FGEN Run.vi"("Instrument Handle In"=w374, "Error In"=w375) -> ("Instrument Handle Out"=w360:refnum<k21>, "Error Out"=w371:errorcluster)  [unwired: 12 in]
        n85 = call "[Scope] Set Sample Rate(Slew Rate).vi"("Frequency"=w327) -> ("Acquistion Time"=w329:dbl, "Sample Rate"=w330:dbl)  [unwired: 9 in]
        n86 = call-poly <vilib>:"MSO Configure Analog Channel.vi"("Instrument Handle In"=w359, "Channel"="Channel", "Error In"=w371, "Vertical Range"="Vertical Range") -> ("Instrument Handle Out"=w368:refnum<k21>, "Error Out"=w369:errorcluster)  [unwired: 10 in]
        n87 = call-poly <vilib>:"MSO Configure Timing.vi"("Instrument Handle In"=w368, "Sample Rate"=w330, "Acquisition Time (s)"=w329, "Error In"=w369) -> ("Instrument Handle Out"=w367:refnum<k21>, "Error Out"=w366:errorcluster)  [unwired: 10 in]
        n88 = case shown="\"Analog Trigger\"" "Trigger Type" {
          tunnel: w367 -> [w382 w385 w390 w400]
          tunnel: w366 -> [w380 w387 w395 w398]
          tunnel: [w381 w384 w391 w401] -> w364
          tunnel: [w379 w388 w394 w402] -> w365
          frame "Immediate Trigger", Default {
            # "Configure Immediate Trigger"
            n89 = call <vilib>:"MSO Configure Immediate Trigger.vi"("Instrument Handle In"=w382, "Error In"=w380) -> ("Instrument Handle Out"=w381:refnum<k21>, "Error Out"=w379:errorcluster)  [unwired: 12 in]
          }
          frame "Digital Trigger" {
            # "Configure Digital Trigger"
            n90 = call-poly <vilib>:"MSO Configure Digital Edge Trigger.vi"("Instrument Handle In"=w385, "Trigger Source"="Digital Trigger Source", "Trigger Slope"="Edge", "Error In"=w387) -> ("Instrument Handle Out"=w384:refnum<k21>, "Error Out"=w388:errorcluster)  [unwired: 10 in]
          }
          frame "Analog Trigger" {
            # "Configure Analog Trigger"
            n91 = call-poly <vilib>:"MSO Configure Analog Edge Trigger.vi"("Instrument Handle In"=w390, "Trigger Hysteresis"="Hysteresis (V)", "Trigger Source"="Analog Trigger Source", "Trigger Slope"="Slope", "Trigger Level"="Level (V)", "Error In"=w395) -> ("Instrument Handle Out"=w391:refnum<k21>, "Error Out"=w394:errorcluster)  [unwired: 8 in]
          }
          frame "Pattern Trigger" {
            # "Configure Pattern Trigger"
            n92 = call-poly <vilib>:"MSO Configure Digital Pattern Trigger.vi"("Instrument Handle In"=w400, "Trigger Source"="Pattern Trigger Source", "Trigger Pattern"="Trigger Pattern", "Error In"=w398) -> ("Instrument Handle Out"=w401:refnum<k21>, "Error Out"=w402:errorcluster)  [unwired: 10 in]
          }
        }
        n93 = call <vilib>:"MSO Run.vi"("Instrument Handle In"=w364, "Error In"=w365) -> ("Instrument Handle Out"=w358:refnum<k21>, "Error Out"=w357:errorcluster)  [unwired: 12 in]
        n94 = call <vilib>:"MSO Read.vi"("Instrument Handle In"=w358, "Error In"=w357) -> ("Instrument Handle Out"=w332:refnum<k21>, "Analog Waveforms"=w338:waveform(dbl)[], "Error Out"=w337:errorcluster)  [unwired: 8 in, 3 out]
        n95 = call <vilib>:"MSO Stop.vi"("Instrument Handle In"=w332, "Error In"=w337) -> ("Instrument Handle Out"=w331:refnum<k21>, "Error Out"=w333:errorcluster)  [unwired: 12 in]
        n96 = call "BW.vi"("错误输入（无错误）"=w333, "frequency"=w327, "Analog Waveforms"=w338) -> ("错误输出"=w340:errorcluster, "Gain Display"=→"Amplitude-frequency":cluster{dbl[], dbl[]})  [unwired: 7 in]
        n97 = Wait (ms)(milliseconds to wait=u32 100 ("等待时间（毫秒）")) -> ()  [unwired: 1 out]
      }
    }
    n98 = local write "测试进度"(w49) -> ()
    n99 = Or(x=w48, y=w47) -> (x .or. y?=w46:bool)
  }
  n100 = call <vilib>:"DWF Dig Close.vi"("Instrument Handle In"=w1, "Error In"=w2) -> ("Error Out"=w3:errorcluster)  [unwired: 13 in]
  n101 = call <vilib>:"Dig Close.vi"("Instrument Handle In"=w19, "Error In"=w3) -> ("Error Out"=w11:errorcluster)  [unwired: 13 in]
  n102 = call <vilib>:"PS Close.vi"("Instrument Handle In"=w20, "Error In"=w11) -> ("Error Out"=w10:errorcluster)  [unwired: 13 in]
  n103 = call <vilib>:"FGEN Close.vi"("Instrument Handle In"=w18, "Error In"=w10) -> ("Error Out"=w9:errorcluster)  [unwired: 13 in]
  n104 = call <vilib>:"DMM Close.vi"("Instrument Handle In"=w21, "Error In"=w9) -> ("Error Out"=w8:errorcluster)  [unwired: 13 in]
  n105 = call <vilib>:"MSO Close.vi"("Instrument Handle In"=w17, "Error In"=w8) -> ("Error Out"=w7:errorcluster)  [unwired: 13 in]
  n106 = case shown="无错误" w7 {
    selector: w7 -> [_ w404]
    frame No Error {
      n107 = local write "测试进度"(u8 100 ("测试进度")) -> ()
    }
    frame Error {
      w405 = T8 3 items=["no dialog", "OK message", "continue or stop message", "OK message + warnings", "continue/stop + warnings"] ("type of dialog (OK msg:1)")
      n108 = call <vilib>:"Simple Error Handler.vi"("type of dialog (OK msg:1)"=w405, "error in (no error)"=w404) -> ()  [unwired: 3 in, 5 out]
    }
  }
